vi "Cal RHS (Numeric).vi"(8 "error in (no error)":errorcluster, 10 "RHS in":variant, 11 "Domain_Evolut_1D in":refnum<class "NI_Domain_Evolut_1D.lvclass">) -> (0 "error out":errorcluster, 2 "RHS out":variant, 3 "Domain_Evolut_1D out":refnum<class "NI_Domain_Evolut_1D.lvclass">)   [LabVIEW 2020, in "NI_PDE.lvlib" / "NI_Domain_Evolut_1D.lvclass"]
uses:
  <vilib>/gmath/pde.llb/DomainClass/Domain_Evolut_1D/NI_Domain_Evolut_1D.lvclass
  <vilib>/gmath/pde.llb/DomainClass/Domain_Evolut_1D/NI_Domain_Evolut_1D.lvclass/NI_Domain_Evolut_1D.ctl
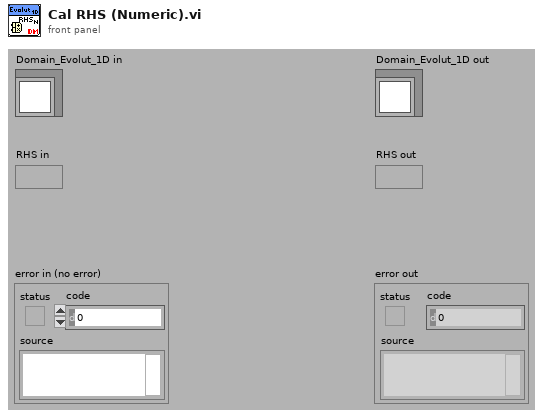
[diagram p1: front panel]
types:
  T1 = cluster{"initial t":dbl, "final t":dbl, "# of t-points":i32}
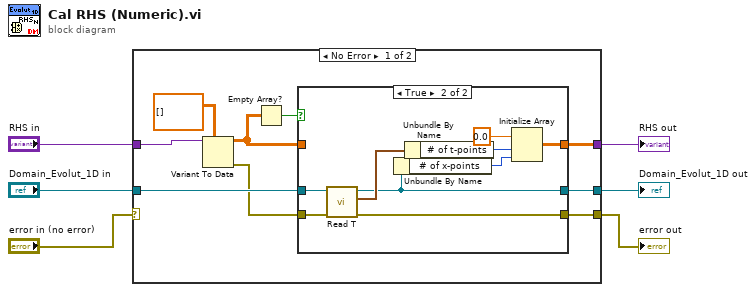
[diagram p0: block diagram]
diagram:
  n1 = case shown="No Error" "error in (no error)" {
    selector: "error in (no error)" -> [_ w30]
    tunnel: "Domain_Evolut_1D in" -> [w14 w28]
    tunnel: [w8 w30] -> w6
    tunnel: [w7 w29] -> w3
    tunnel: "RHS in" -> [w11 w29]
    tunnel: [w9 w28] -> w1
    frame No Error {
      n2 = Variant To Data(type=dbl[][] [] ("F"), Variant=w11) -> (data=w12:dbl[][], error out=w10:errorcluster)  [unwired: 1 in]
      n3 = Empty Array?(array=w12) -> (empty?=w15:bool)
      n4 = case shown="True" w15 {
        tunnel: w14 -> [w16 w22]
        tunnel: w12 -> [w18 _]
        tunnel: [w17 w23] -> w8
        tunnel: [w18 w26] -> w7
        tunnel: w10 -> [w17 w21]
        tunnel: [w16 w19] -> w9
        frame False {
        }
        frame True {
          n5 = call-dynamic "Read T.vi"("error in (no error)"=w21, "Domain_Evolut.lvclass in"=w22) -> ("error out"=w23:errorcluster, "t"=w20:T1, "Domain_Evolut.lvclass out"=w19:refnum<class "NI_Domain_Evolut_1D.lvclass">)  [unwired: 7 out]
          n6 = Unbundle By Name(w19) -> ("# of x-points"=w24:i32)
          n7 = Unbundle By Name(w20) -> ("# of t-points"=w27:i32)
          n8 = Initialize Array(0.0 ("element"), w27, w24) -> (w26:dbl[][])
        }
      }
    }
    frame Error {
    }
  }
  "Domain_Evolut_1D out" <- w1
  "error out" <- w6
  "RHS out" <- w3
